vi "DSF.Engine.Transfer Group.Set Engine Offset.vi"(10 "engine offset":u64, 11 "Transfer Group in":refnum<class "DSF.Engine.Transfer Group.lvclass">) -> (3 "Transfer Group out":refnum<class "DSF.Engine.Transfer Group.lvclass">)   [LabVIEW 2017, in "DSF.Engine.lvlib" / "DSF.Engine.Transfer Group.lvclass"]
uses:
  DSF.Engine.Transfer Group.lvclass
  DSF.Engine.Transfer Group.lvclass/DSF.Engine.Transfer Group.ctl
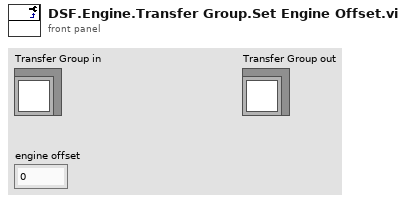
[diagram p1: front panel]
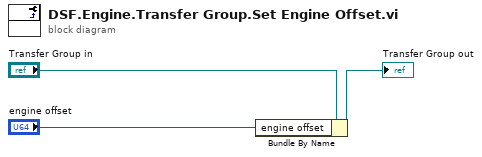
[diagram p0: block diagram]
diagram:
  n1 = Bundle By Name(cluster="Transfer Group in", "engine offset"="engine offset") -> (→"Transfer Group out":refnum<class "DSF.Engine.Transfer Group.lvclass">)
